vi "How to generate fibonacci series.vi"() -> ()   [LabVIEW 2020]
panel:
  in  "OK Button":bool
  in  "stop":bool
  out "Numeric 2":dbl
  in  "Numeric":dbl
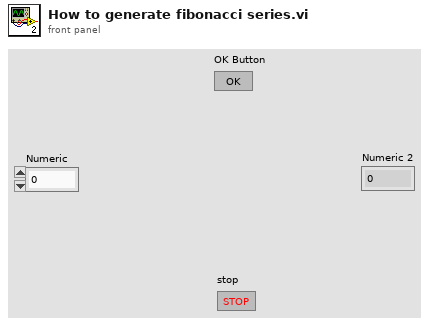
[diagram p1: front panel]
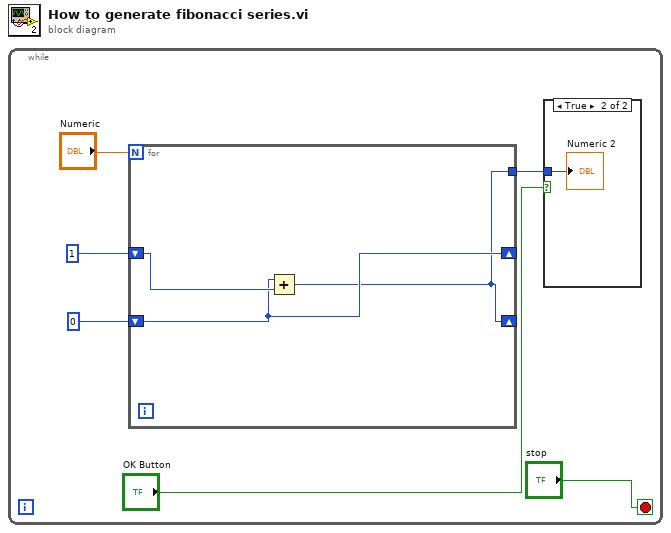
[diagram p0: block diagram]
diagram:
  n1 = while {
    stop <- "stop" stop-if-true
    n2 = for {
      N: "Numeric" -> [_]
      shift-right: [w9] -> _
      shift-left: 1 -> [w10]
      shift-right: [w8] -> _
      shift-left: 0 -> [w9]
      tunnel: [w8] -> w3
      n3 = Add(x=w9, y=w10) -> (x+y=w8:i32)
    }
    n4 = case shown="True" "OK Button" {
      tunnel: w3 -> [_ w7]
      frame False {
      }
      frame True {
        "Numeric 2" <- w7
      }
    }
  }
